vi "Set Message Data.vi"(8 "error in":errorcluster, 10 "Enum values":string, 11 "Control ref in":refnum<vi>) -> (0 "error out":errorcluster, 3 "Control ref out":refnum<vi>)   [LabVIEW 2019, in "gRPC Template Creation Utility.lvlib"]
uses:
  gRPC Template Creation Utility.lvlib
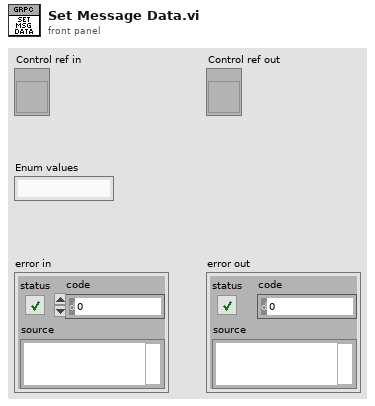
[diagram p1: front panel]
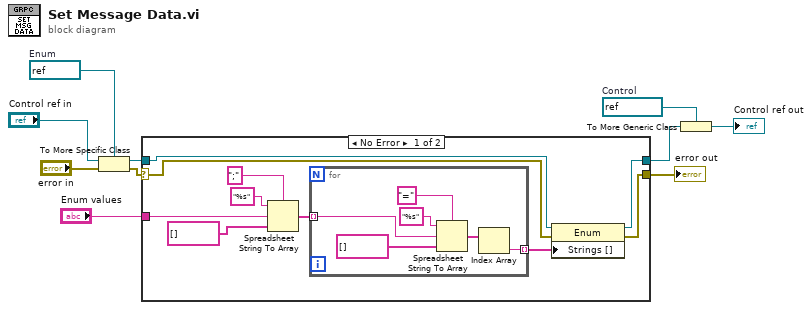
[diagram p0: block diagram]
diagram:
  w2 = refnum<vi> refnum  # Control
  w5 = refnum<vi> refnum  # Enum
  n1 = To More Specific Class(target class=w5, reference="Control ref in", error in="error in") -> (specific class reference=w4:refnum<vi>, error out=w3:errorcluster)
  n2 = case shown="No Error" w3 {
    selector: w3 -> [w16 w28]
    tunnel: w4 -> [w20 w27]
    tunnel: "Enum values" -> [w19 _]
    tunnel: [w17 w28] -> w7
    tunnel: [w13 w27] -> w1
    frame No Error {
      n3 = Spreadsheet String To Array(delimiter (Tab)=";", format string="%s", spreadsheet string=w19, array type (2D Dbl)=string[] []) -> (array=w12:string[])
      n4 = for {
        tunnel: w12 -> [w22] mode=indexing
        tunnel: [w21] -> w11 mode=indexing
        n5 = Spreadsheet String To Array(delimiter (Tab)="=", format string="%s", spreadsheet string=w22, array type (2D Dbl)=string[] []) -> (array=w23:string[])
        n6 = Index Array(array=w23) -> (element=w21:string)  [unwired: 1 in]
      }
      n7 = property class="Enum"(reference=w20, error in=w16, "Strings []"=w11) -> (reference out=w13:refnum<vi>, error out=w17:errorcluster)
    }
    frame Error {
    }
  }
  "error out" <- w7
  n8 = To More Generic Class(target class=w2, reference=w1) -> (generic class reference=→"Control ref out":refnum<vi>)
